vi "exampleMQTT_Client.vi"() -> ()   [LabVIEW 2023]
uses:
  <vilib>/LabVIEW Open Source Project/MQTT Client/Client class/Client.lvclass/Client.ctl
  <vilib>/LabVIEW Open Source Project/MQTT Connection/MQTT_Base/Base Class/MQTT_Base.lvclass/MQTT_Base.ctl
  <vilib>/LabVIEW Open Source Project/MQTT Control Packets/Control Packets/ControlPacket/ControlPacket.lvclass/ControlPacket.ctl
  <vilib>/LabVIEW Open Source Project/Connection/Connection.TCP/Connection.TCP.lvclass
  C:/Program Files (x86)/National Instruments/LabVIEW 2023/vi.lib/LabVIEW Open Source Project/Connection/Connection/Connection.lvclass
  <vilib>/LabVIEW Open Source Project/MQTT Client/Client class/Client.lvclass
  C:/Program Files (x86)/National Instruments/LabVIEW 2023/vi.lib/LabVIEW Open Source Project/MQTT Connection/MQTT_Base/Base Class/MQTT_Base.lvclass
  <vilib>/LabVIEW Open Source Project/MQTT Control Packets/Control Packets/PUBLISH/PUBLISH.lvclass
  C:/Program Files (x86)/National Instruments/LabVIEW 2023/vi.lib/LabVIEW Open Source Project/MQTT Control Packets/Control Packets/ControlPacket/ControlPacket.lvclass
  <vilib>/LabVIEW Open Source Project/MQTT Connection/MQTT_Base/Base Class/MQTT_Base.lvclass
  <vilib>/LabVIEW Open Source Project/MQTT Control Packets/Control Packets/ControlPacket/ControlPacket.lvclass
  <vilib>/LabVIEW Open Source Project/Connection/Connection.LocalQueue/Connection.LocalQueue.lvclass
  <vilib>/LabVIEW Open Source Project/Connection/Connection/Connection.lvclass
panel:
  out "Incoming Message":u8[](array[numeric]) format="%08b"
  in  "Subscribe":bool
  out "Suback":bool
  out "Published":bool
  in  "Publish":bool
  in  "Stop Client":bool
  out "error out":errorcluster
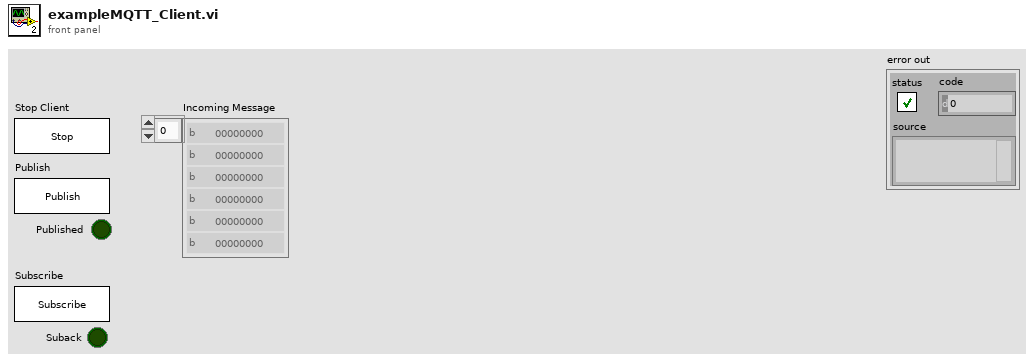
[diagram p1: front panel]
types:
  T1 = typedef "MQTT Client.lvlib/Client.lvclass/Public Events -- cluster.ctl" = cluster{"Connection Status":refnum<user-event>, "Connected":refnum<user-event>, "Application Message":refnum<user-event>}
  T2 = typedef "MQTT Base.lvlib/MQTT_Base.lvclass/Public Events -- cluster.ctl" = cluster{"Stop Event":refnum<user-event>, "Error Event":refnum<user-event>, "Inbound Message":refnum<user-event>}
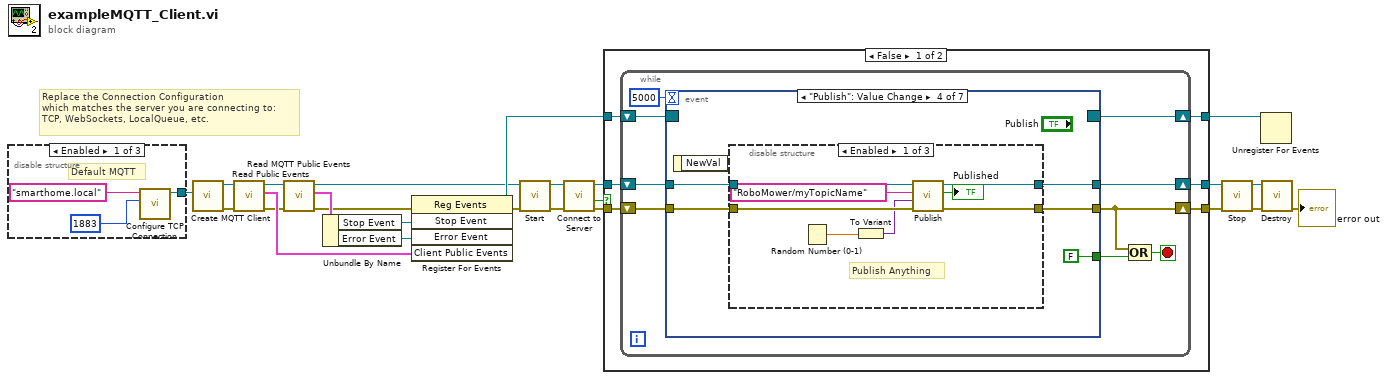
[diagram p0: block diagram]
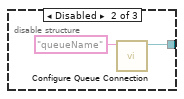
[diagram p2: hidden frame]
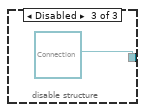
[diagram p3: hidden frame]
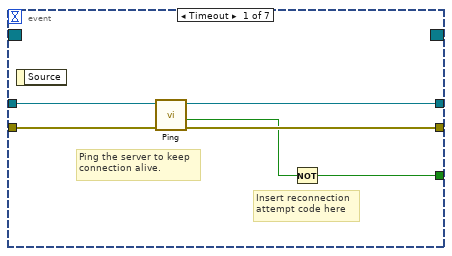
[diagram p4: hidden frame]
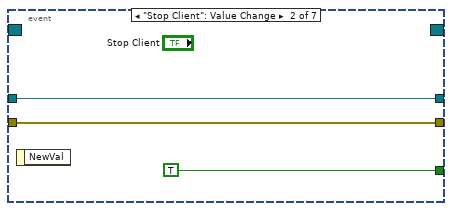
[diagram p5: hidden frame]
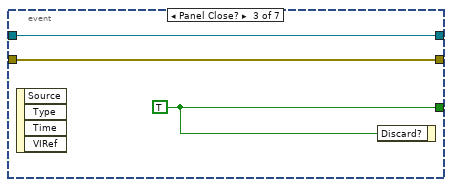
[diagram p6: hidden frame]
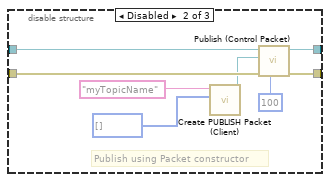
[diagram p7: hidden frame]
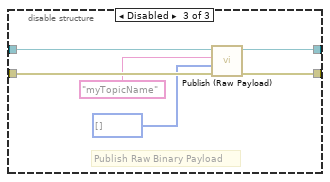
[diagram p8: hidden frame]
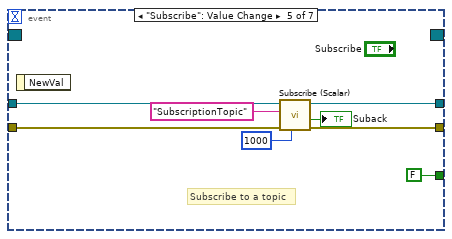
[diagram p9: hidden frame]
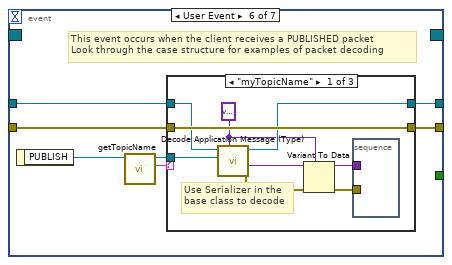
[diagram p10: hidden frame]
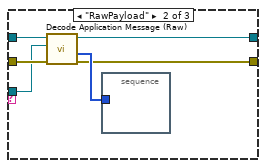
[diagram p11: hidden frame]
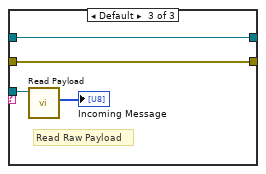
[diagram p12: hidden frame]
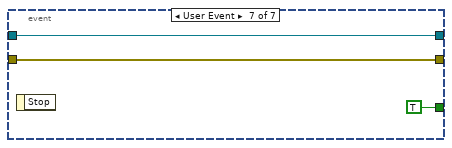
[diagram p13: hidden frame]
diagram:
  # "Replace the Connection Configuration\nwhich matches the server you are connecting to:\nTCP, WebSockets, LocalQueue, etc."
  n1 = disable-structure shown="Enabled" {
    disable-tunnel: [w26 w29 refnum<class "Connection.lvclass"> refnum ("Connection Configuration")] -> w24
    frame Enabled {
      # "Default MQTT"
      n2 = call <vilib>:"Configure TCP Connection.vi"("remote port (80)"=u16 1883, "address (localhost)"="smarthome.local") -> ("Connection.TCP"=w26:refnum<class "Connection.TCP.lvclass">)  [unwired: 8 in, 1 out]
    }
    frame Disabled {
      n3 = call <vilib>:"Configure Queue Connection.vi"("Queue Name"="queueName") -> ("Connection.LocalQueue"=w29:refnum<class "Connection.LocalQueue.lvclass">)  [unwired: 9 in, 1 out]
    }
    frame Disabled {
    }
  }
  n4 = call <vilib>:"Create MQTT Client.vi"("Connection Configuration"=w24) -> ("error out"=w3:errorcluster, "Client out"=w1:refnum<class "Client.lvclass">)  [unwired: 9 in]
  n5 = call <vilib>:"Read Public Events.vi"("error in (no error)"=w3, "Client in"=w1) -> ("error out"=w4:errorcluster, "Client Public Events"=w6:T1, "Client out"=w2:refnum<class "Client.lvclass">)  [unwired: 7 in]
  n6 = call <vilib>:"Read MQTT Public Events.vi"("error in (no error)"=w4, "MQTT_Base in"=w2) -> ("error out"=w5:errorcluster, "MQTT Public Events"=w18:T2, "MQTT_Base out"=w8:refnum<class "Client.lvclass">)  [unwired: 7 in]
  n7 = Unbundle By Name(w18) -> ("Stop Event"=w16:refnum<user-event>, "Error Event"=w17:refnum<user-event>)
  n8 = register-events(error in=w5, w16, w17, w6) -> (reference out=w11:refnum<event-registration>, error out=w7:errorcluster)  [unwired: 1 in]
  n9 = call <vilib>:"Start.vi"("error in (no error)"=w7, "MQTT_Base in"=w8) -> ("error out"=w10:errorcluster, "MQTT_Base out"=w9:refnum<class "Client.lvclass">)  [unwired: 7 in, 1 out]
  n10 = call <vilib>:"Connect to Server.vi"("error in (no error)"=w10, "Client in"=w9) -> ("error out"=w14:errorcluster, "timed out"=w13:bool, "Client out"=w15:refnum<class "Client.lvclass">)  [unwired: 6 in, 1 out]
  n11 = case shown="False" w13 {
    tunnel: w11 -> [w36 w124]
    tunnel: [w35 w124] -> w12
    tunnel: w14 -> [w32 w122]
    tunnel: w15 -> [w34 w123]
    tunnel: [w33 w123] -> w20
    tunnel: [w31 w122] -> w22
    frame False {
      n12 = while {
        shift-right: [w44] -> w35
        shift-left: w36 -> [w45]
        shift-right: [w37] -> w33
        shift-left: w34 -> [w38]
        shift-right: [w42] -> w31
        shift-left: w32 -> [w43]
        stop <- w41 stop-if-true
        n13 = event shown="[3] \"Publish\": Value Change" {
          selector: w45 -> [_ _ _ _ _ _ _]
          dyn-events: [_ _ _ _ _ _ _] -> w44
          timeout: 5000 -> [_ _ _ _ _ _ _]
          tunnel: w43 -> [w50 w53 w55 w60 w89 w94 w121]
          tunnel: [w48 w53 w55 w59 w88 w95 w121] -> w42
          tunnel: [w47 TRUE w57 FALSE FALSE _ TRUE] -> w40
          tunnel: w38 -> [w51 w54 w56 w61 w91 w97 w119]
          tunnel: [w49 w54 w56 w58 w87 w96 w119] -> w37
          event Timeout {
            # "Insert reconnection\nattempt code here"
            # "Ping the server to keep\nconnection alive."
            n14 = event-data() -> ()  [unwired: 1 in, 1 out]
            n15 = call <vilib>:"Ping.vi"("error in (no error)"=w50, "Client in"=w51) -> ("error out"=w48:errorcluster, "Server responded"=w46:bool, "Client out"=w49:refnum<class "Client.lvclass">)  [unwired: 6 in, 1 out]
            n16 = Not(x=w46) -> (.not. x?=w47:bool)
          }
          event "Stop Client": Value Change {
            n17 = event-data() -> ()  [unwired: 1 in, 1 out]
          }
          event Panel Close? {
            w57 = TRUE
            n18 = event-data() -> ()  [unwired: 1 in, 4 out]
            n19 = event-data("Discard?"=w57) -> ()  [unwired: 1 in, 1 out]
          }
          event "Publish": Value Change {
            n20 = event-data() -> ()  [unwired: 1 in, 1 out]
            n21 = disable-structure shown="Enabled" {
              disable-tunnel: w61 -> [w70 w76 w84]
              disable-tunnel: w60 -> [w69 w74 w81]
              disable-tunnel: [w68 w73 w82] -> w59
              disable-tunnel: [w67 w75 w83] -> w58
              frame Enabled {
                # "Publish Anything"
                n22 = Random Number (0-1)() -> (number: 0 to 1=w65:dbl)
                n23 = To Variant(anything=w65) -> (Variant=w64:variant)
                n24 = call <vilib>:"Publish.vi"("error in (no error)"=w69, "Payload"=w64, "Topic Name (empty: Payload name)"="RoboMower/myTopicName", "Client in"=w70) -> ("error out"=w68:errorcluster, "Published"=→"Published":bool, "Client out"=w67:refnum<class "Client.lvclass">)  [unwired: 5 in]
              }
              frame Disabled {
                # "Publish using Packet constructor"
                n25 = call <vilib>:"Create PUBLISH Packet (Client).vi"("Payload"=u8[] [], "Topic Name"="myTopicName" ("Topic Name (empty: Payload name)")) -> ("PUBLISH"=w71:refnum<class "PUBLISH.lvclass">)  [unwired: 6 in, 3 out]
                n26 = call <vilib>:"Publish (Control Packet).vi"("timeout (1000ms)"=100 ("timeout (0ms : no ack)"), "error in (no error)"=w74, "PUBLISH"=w71, "Client in"=w76) -> ("error out"=w73:errorcluster, "Client out"=w75:refnum<class "Client.lvclass">)  [unwired: 5 in, 1 out]
              }
              frame Disabled {
                # "Publish Raw Binary Payload"
                n27 = call <vilib>:"Publish (Raw Payload).vi"("error in (no error)"=w81, "Binary Payload"=u8[] [] ("Payload"), "Topic Name"="myTopicName" ("Topic Name (empty: Payload name)"), "Client in"=w84) -> ("error out"=w82:errorcluster, "Client out"=w83:refnum<class "Client.lvclass">)  [unwired: 5 in, 1 out]
              }
            }
          }
          event "Subscribe": Value Change {
            # "Subscribe to a topic"
            n28 = event-data() -> ()  [unwired: 1 in, 1 out]
            n29 = call <vilib>:"Subscribe (Scalar).vi"("timeout (1000ms)"=1000 ("timeout (100ms)"), "error in (no error)"=w89, "Topic Filter"="SubscriptionTopic" ("Topic Name (empty: Payload name)"), "Client in"=w91) -> ("error out"=w88:errorcluster, "Ack"=→"Suback":bool, "Client out"=w87:refnum<class "Client.lvclass">)  [unwired: 5 in]
          }
          event User Event {
            # "This event occurs when the client receives a PUBLISHED packet\nLook through the case structure for examples of packet decoding"
            n30 = event-data() -> ("PUBLISH"=w99:refnum<class "PUBLISH.lvclass">)  [unwired: 1 in]
            n31 = call <vilib>:"getTopicName.vi"("PUBLISH in"=w99) -> ("Topic"=w98:string, "PUBLISH out"=w93:refnum<class "PUBLISH.lvclass">)  [unwired: 8 in, 1 out]
            n32 = case shown="\"myTopicName\"" w98 {
              tunnel: w97 -> [w105 w114 w118]
              tunnel: [w104 w113 w118] -> w96
              tunnel: [w108 w111 w117] -> w95
              tunnel: w94 -> [w108 w110 w117]
              tunnel: w93 -> [w103 w109 w116]
              frame "myTopicName" {
                w101 = variant ("Type")
                # "Use Serializer in the\nbase class to decode"
                n33 = call <vilib>:"Decode Application Message (Type).vi"("Type"=w101, "PUBLISH"=w103, "Client in"=w105) -> ("error out"=w100:errorcluster, "Payload"=w102:variant, "Client out"=w104:refnum<class "Client.lvclass">)  [unwired: 5 in, 1 out]
                n34 = Variant To Data(error in=w100, type=w101, Variant=w102) -> (data=w107:variant, error out=w106:errorcluster)
                n35 = stacked-sequence {
                  tunnel: w107 -> [_]
                  tunnel: w106 -> [_]
                  frame #0 {
                  }
                }
              }
              frame "RawPayload" {
                n36 = call <vilib>:"Decode Application Message (Raw).vi"("error in (no error)"=w110, "PUBLISH"=w109, "Client in"=w114) -> ("error out"=w111:errorcluster, "Payload"=w112:u8[], "Client out"=w113:refnum<class "Client.lvclass">)  [unwired: 5 in, 1 out]
                n37 = stacked-sequence {
                  tunnel: w112 -> [_]
                  frame #0 {
                  }
                }
              }
              frame Default {
                # "Read Raw Payload"
                n38 = call <vilib>:"Read Payload.vi"("ControlPacket in"=w116) -> ("Payload"=→"Incoming Message":u8[])  [unwired: 9 in, 1 out]
              }
            }
          }
          event User Event {
            n39 = event-data() -> ()  [unwired: 1 in, 1 out]
          }
        }
        n40 = Compound Arithmetic op=OR(w42, w40) -> (w41:bool)
      }
    }
    frame True {
    }
  }
  n41 = call <vilib>:"Stop.vi"("error in (no error)"=w22, "MQTT_Base in"=w20) -> ("error out"=w21:errorcluster, "MQTT_Base out"=w19:refnum<class "Client.lvclass">)  [unwired: 7 in, 1 out]
  n42 = Unregister For Events(event registration refnum=w12) -> ()  [unwired: 1 in, 1 out]
  n43 = call <vilib>:"Destroy.vi"("error in (no error)"=w21, "MQTT_Base in"=w19) -> ("error out"=→"error out":errorcluster)  [unwired: 8 in, 1 out]
